vi "Select Color to Display.vi"(8 "error in (no error)":errorcluster, 11 "GameLogic in":refnum<class "GameLogic.lvclass">) -> (0 "error out":errorcluster, 3 "GameLogic out":refnum<class "GameLogic.lvclass">)   [LabVIEW 2019, in "GameLogic.lvlib" / "GameLogic.lvclass"]
uses:
  GameLogic.lvclass
  C:/Program Files (x86)/National Instruments/LabVIEW 2019/vi.lib/ActorFramework/Actor/Actor.lvclass
  GameLogic.lvclass/GameLogic.ctl
  <vilib>/ActorFramework/Actor/Actor.lvclass/Actor.ctl
  <vilib>/ActorFramework/Message Enqueuer/Message Enqueuer.lvclass/Message Enqueuer.ctl
  <vilib>/ActorFramework/Message Enqueuer/Init from Existing Queue.vi
  <vilib>/ActorFramework/Message Enqueuer/Enqueue.vi
  GameLogic Messages/Display Color Sequence Msg/Display Color Sequence Msg.lvclass
  C:/Program Files (x86)/National Instruments/LabVIEW 2019/vi.lib/ActorFramework/Message/Message.lvclass
  GameLogic Messages/Turn all Colors off Msg/Turn all Colors off Msg.lvclass
  <vilib>/ActorFramework/Message Priority Queue/Priority Enqueue.vi
  <userlib>/_MGI/Timing/MGI Wait/MGI Wait (U32).vi
  <vilib>/ActorFramework/Message Enqueuer/Message Enqueuer.lvclass
  <vilib>/ActorFramework/Actor/Actor.lvclass
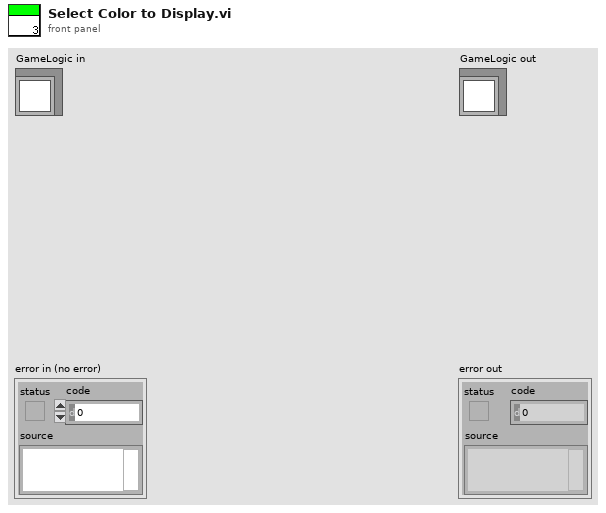
[diagram p1: front panel]
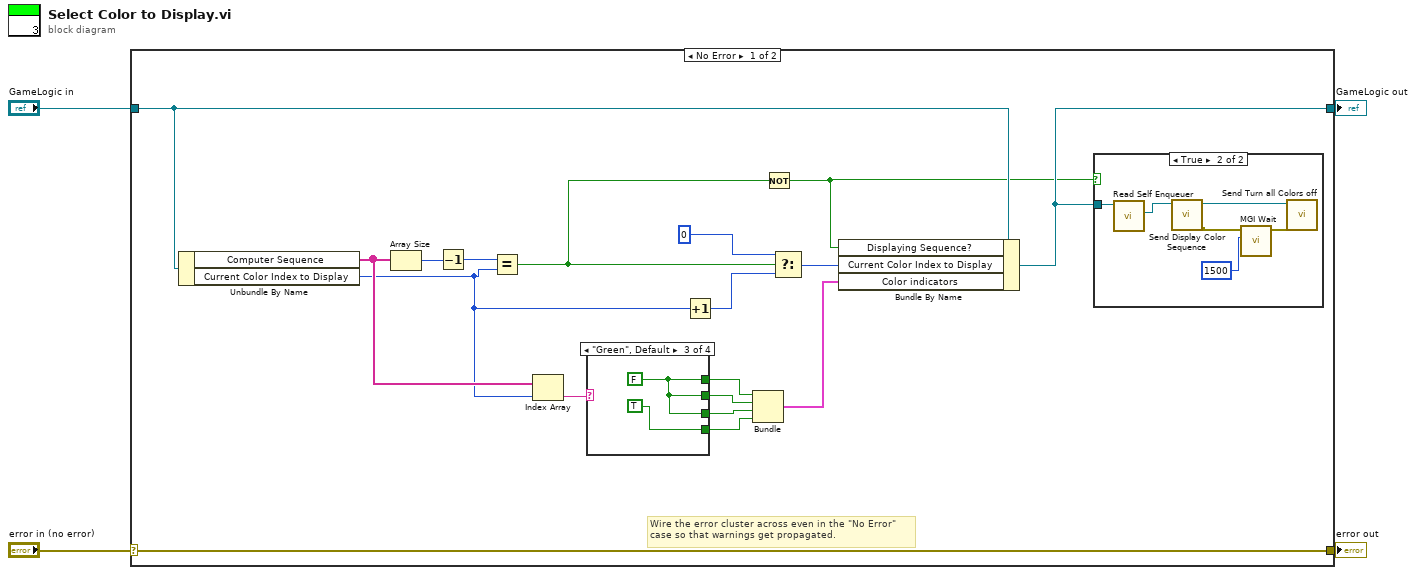
[diagram p0: block diagram]
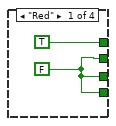
[diagram p3: hidden frame]
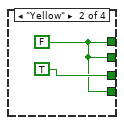
[diagram p4: hidden frame]
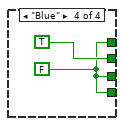
[diagram p5: hidden frame]
diagram:
  n1 = case shown="No Error" "error in (no error)" {
    selector: "error in (no error)" -> [w22 w38]
    tunnel: [w22 w38] -> w3
    tunnel: [w6 w37] -> w1
    tunnel: "GameLogic in" -> [w7 w37]
    frame No Error {
      # "Wire the error cluster across even in the \"No Error\"\ncase so that warnings get propagated."
      n2 = Unbundle By Name(w7) -> ("Computer Sequence"=w11:string[], "Current Color Index to Display"=w10:i32)
      n3 = Array Size(array=w11) -> (size(s)=w20:i32)
      n4 = Decrement(x=w20) -> (x-1=w19:i32)
      n5 = Equal?(x=w19, y=w10) -> (x = y?=w12:bool)
      n6 = Index Array(array=w11, index=w10) -> (element=w21:string)
      n7 = case shown="\"Green\", Default" w21 {
        tunnel: [TRUE w31 w33 w35] -> w18
        tunnel: [w29 w31 w33 TRUE] -> w17
        tunnel: [w29 TRUE w33 w35] -> w16
        tunnel: [w29 w31 TRUE w35] -> w15
        frame "Red" {
          w29 = FALSE
        }
        frame "Yellow" {
          w31 = FALSE
        }
        frame "Green", Default {
          w33 = FALSE
        }
        frame "Blue" {
          w35 = FALSE
        }
      }
      n8 = Increment(x=w10) -> (x+1=w14:i32)
      n9 = Bundle(w18, w17, w16, w15) -> (w8:cluster{bool, bool, bool, bool})  [unwired: 1 in]
      n10 = Not(x=w12) -> (.not. x?=w5:bool)
      n11 = Select(t=0, s=w12, f=w14) -> (s? t:f=w9:i32)
      n12 = Bundle By Name(cluster=w7, "Displaying Sequence?"=w5, "Current Color Index to Display"=w9, "Color indicators"=w8) -> (w6:refnum<class "GameLogic.lvclass">)
      n13 = case shown="True" w5 {
        tunnel: w6 -> [_ w28]
        frame False {
        }
        frame True {
          n14 = call <vilib>:"Read Self Enqueuer.vi"("Actor"=w28) -> ("Self Enqueuer"=w27:refnum<class "Message Enqueuer.lvclass">)  [unwired: 10 in]
          n15 = call "Send Display Color Sequence.vi"("Message Enqueuer"=w27) -> ("error out"=w24:errorcluster, "Message Enqueuer out"=w26:refnum<class "Message Enqueuer.lvclass">)  [unwired: 9 in]
          n16 = call-poly <userlib>:"MGI Wait.vi"("ms"=u32 1500, "Error In"=w24) -> ("Error Out"=w23:errorcluster)  [unwired: 5 in]
          n17 = call "Send Turn all Colors off.vi"("error in (no error)"=w23, "Message Enqueuer"=w26) -> ()  [unwired: 8 in, 2 out]
        }
      }
    }
    frame Error {
    }
  }
  "error out" <- w3
  "GameLogic out" <- w1
